vi "DiffDrivePoseEst2_Execute.vi"(0 "Vision TImeStamp_Seconds":dbl=0.02, 3 "TrackWidth_Meters":dbl=1.2 format="%#_13g", 4 "visionRobotPose":T1={"TRANSLATION"={"X"=0.0, "Y"=0.0}, "ROTATION"={"VALUE"=0.0, "COS"=1.0, "SIN"=0.0}} {"ROTATION"."SIN" format="%13.4f"; "ROTATION"."COS" format="%13.4f"; "ROTATION"."VALUE" format="%13.4f"; "TRANSLATION"."Y" format="%14.3f"; "TRANSLATION"."X" format="%14.3f"}, 5 "Game Started":bool, 6 "Add Vision Meas":bool, 7 "InitialPose":T1={"TRANSLATION"={"X"=0.0, "Y"=0.0}, "ROTATION"={"VALUE"=0.0, "COS"=1.0, "SIN"=0.0}} {"ROTATION"."SIN" format="%13.4f"; "ROTATION"."COS" format="%13.4f"; "ROTATION"."VALUE" format="%13.4f"; "TRANSLATION"."Y" format="%14.3f"; "TRANSLATION"."X" format="%14.3f"}, 8 "Pass Through Time":dbl=-1.0, 9 "Gyro Degrees":dbl, 10 "RightDistance_M":dbl=0.02, 11 "LeftDistance_M":dbl=0.02) -> (1 "Error":bool, 2 "Estimated Pose":T1={"TRANSLATION"={"X"=0.0, "Y"=0.0}, "ROTATION"={"VALUE"=0.0, "COS"=1.0, "SIN"=0.0}} {"ROTATION"."SIN" format="%13.4f"; "ROTATION"."COS" format="%13.4f"; "ROTATION"."VALUE" format="%13.4f"; "TRANSLATION"."Y" format="%14.3f"; "TRANSLATION"."X" format="%14.3f"})   [LabVIEW 2020]
uses:
  <vilib>/Rock Robotics/WPI/ThirdParty/JAS_Junk/TrajLib/TypeDef/POSE2D.ctl
  <vilib>/Rock Robotics/WPI/ThirdParty/JAS_Junk/TrajLib/TypeDef/TRANSLATION2D.ctl
  <vilib>/Rock Robotics/WPI/ThirdParty/JAS_Junk/TrajLib/TypeDef/ROTATION2D.ctl
  <vilib>/Rock Robotics/WPI/ThirdParty/JAS_Junk/TrajLib/Conv_Deg_Radians.vi
  <vilib>/Rock Robotics/WPI/ThirdParty/JAS_Junk/TrajLib/Rotation2d_CreateAngle.vi
  <vilib>/Rock Robotics/WPI/ThirdParty/JAS_Junk/TrajLib/VI/Util_GetTime_U32.vi
  <vilib>/Rock Robotics/SystemInterfaces/NetworkCommunication/NetComm_UsageReport_report.vi
  <vilib>/Rock Robotics/WPI/ThirdParty/JAS_Junk/TrajLib/VI/Util_GetTime_U64.vi
  <vilib>/Rock Robotics/WPI/ThirdParty/JAS_Junk/TrajLib/Globals/Util_LibraryGlobals.vi
  <vilib>/Rock Robotics/WPI/ThirdParty/JAS_Junk/TrajLib/Trajectory_Library.lvlib
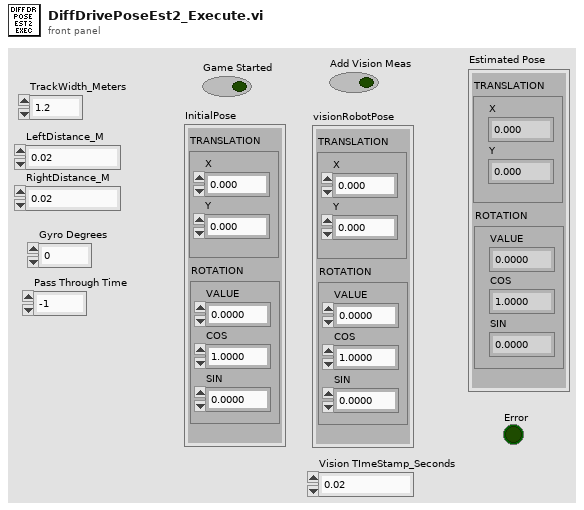
[diagram p1: front panel]
types:
  T1 = typedef "Trajectory_Library.lvlib/POSE2D.ctl" = cluster{"TRANSLATION":T2, "ROTATION":T3}
  T2 = typedef "Trajectory_Library.lvlib/TRANSLATION2D.ctl" = cluster{"X":dbl, "Y":dbl}
  T3 = typedef "Trajectory_Library.lvlib/ROTATION2D.ctl" = cluster{"VALUE":dbl, "COS":dbl, "SIN":dbl}
  T4 = typedef "Trajectory_Library.lvlib/DIFF_DRIVE_KINEMATICS.ctl" = cluster{"TrackWidth_Meters":dbl}
  T5 = typedef "Trajectory_Library.lvlib/DIFF_DRIVE_POSE_EST2.ctl" = cluster{"M_Vision_K":T6, "m_nominal_dT":dbl, "m_PrevTime_Sec":dbl, "Pose_Buffer":T7, "Diff_Drive_Kinematics":T4, "Diff_Drive_Odom_2":T8, "M_Q":T6}
  T6 = typedef "NI_Matrix.lvlib/RealMatrix.ctl" = dbl[][]
  T7 = typedef "Trajectory_Library.lvlib/TIME_INTERPOLATABLE_VARIANT.ctl" = cluster{"TimeStamps":dbl[], "DataArray":variant[], "Min_TimeStamp":dbl, "Max_TimeStamp":dbl, "ItemCount":i32, "MaxBufferTime":dbl}
  T8 = typedef "Trajectory_Library.lvlib/DIFF_DRIVE_ODOM2.ctl" = cluster{"M_POSE_Meters":T1, "M_GyroOffset":T3, "M_PrevAngle":T3, "M_PrevLeftDist_M":dbl, "M_PrevRightDist_M":dbl, "M_InitLeftDist_M":dbl, "M_InitRightDist_M":dbl}
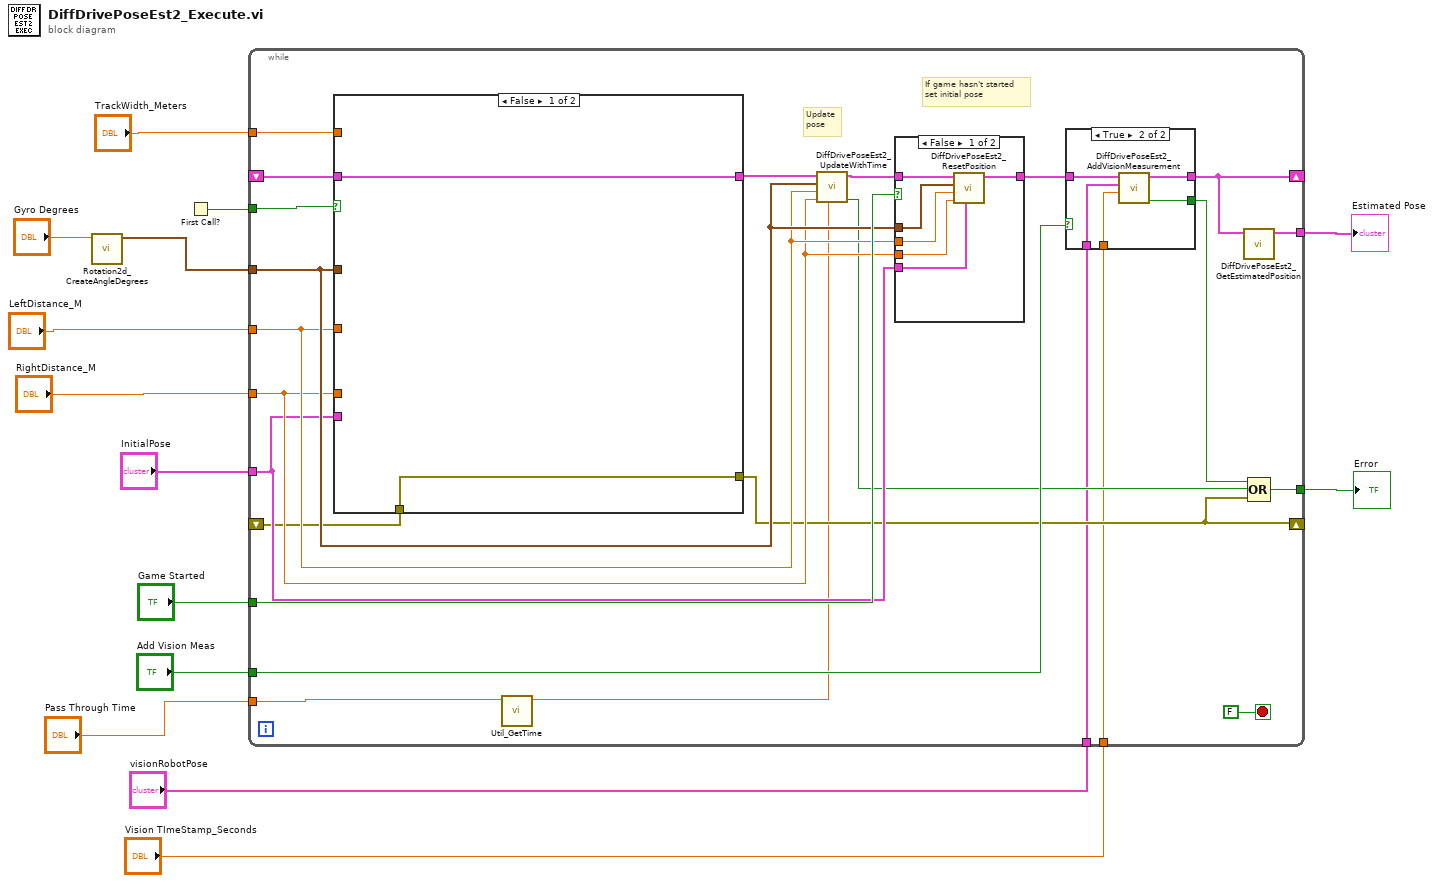
[diagram p0: block diagram]
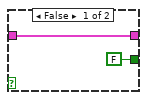
[diagram p3: hidden frame]
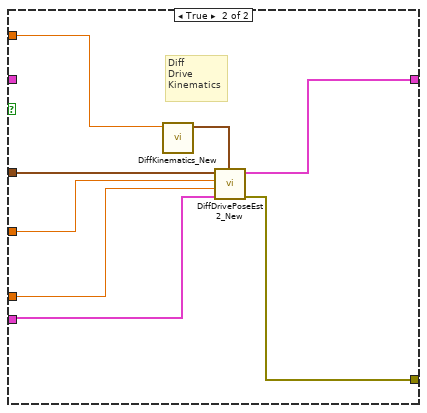
[diagram p4: hidden frame]
diagram:
  n1 = call <vilib>:"Rotation2d_CreateAngleDegrees.vi"("Angle_Degrees"="Gyro Degrees") -> ("ROTATION"=w3:T3)  [unwired: 10 in]
  n2 = First Call?() -> (First Call?: T/F=w14:bool)
  n3 = while {
    tunnel: w14 -> [w37]
    tunnel: w3 -> [w33]
    tunnel: "LeftDistance_M" -> [w32]
    tunnel: "RightDistance_M" -> [w31]
    tunnel: "InitialPose" -> [w30]
    tunnel: "Game Started" -> [w34]
    shift-right: [w23] -> _
    shift-left: _ -> [w28]
    tunnel: "Add Vision Meas" -> [w27]
    shift-right: [w24] -> _
    shift-left: _ -> [w18]
    tunnel: [w22] -> w8
    tunnel: [w21] -> w7
    tunnel: "visionRobotPose" -> [w20]
    tunnel: "Vision TImeStamp_Seconds" -> [w19]
    tunnel: "Pass Through Time" -> [w16]
    tunnel: "TrackWidth_Meters" -> [w15]
    stop <- FALSE stop-if-true
    # "If game hasn't started\nset initial pose"
    # "Update\npose"
    n4 = case shown="False" w37 {
      tunnel: w33 -> [_ w61]
      tunnel: w32 -> [_ w60]
      tunnel: w31 -> [_ w59]
      tunnel: w30 -> [_ w58]
      tunnel: [w53 w57] -> w24
      tunnel: [w54 w56] -> w36
      tunnel: w28 -> [w54 _]
      tunnel: w18 -> [w53 _]
      tunnel: w15 -> [_ w55]
      frame False {
      }
      frame True {
        # "Diff\nDrive\nKinematics"
        n5 = call <vilib>:"DiffKinematics_New.vi"("TrackWidth_Meters"=w55) -> ("DIFF_DRIVE_KINEMATICS"=w62:T4)  [unwired: 10 in]
        n6 = call <vilib>:"DiffDrivePoseEst2_New.vi"("DIFF_DRIVE_KINEMATICS"=w62, "InitialPose"=w58, "RightDistance_M"=w59, "LeftDistance_M"=w60, "gyroAngle"=w61) -> ("Error"=w57:errorcluster, "DiffDrivePoseEstimate"=w56:T5)  [unwired: 5 in]
      }
    }
    n7 = call <vilib>:"Util_GetTime.vi"("Pass_Through_Time"=w16) -> ("FPGA_Time_Seconds"=w17:dbl)  [unwired: 8 in, 2 out]
    n8 = call <vilib>:"DiffDrivePoseEst2_UpdateWithTime.vi"("CurrentTimeSeconds"=w17, "RightDistance"=w31, "LeftDistance"=w32, "GyroAngle"=w33, "in DiffDrivePoseEst2"=w36) -> ("Error"=w26:bool, "Out DiffDrivePoseEst2"=w35:T5)  [unwired: 4 in, 1 out]
    n9 = case shown="False" w34 {
      tunnel: w35 -> [w44 w45]
      tunnel: w33 -> [w43 _]
      tunnel: w32 -> [w42 _]
      tunnel: w31 -> [w41 _]
      tunnel: w30 -> [w40 _]
      tunnel: [w39 w45] -> w29
      frame False {
        n10 = call <vilib>:"DiffDrivePoseEst2_ResetPosition.vi"("Pose"=w40, "RightDistance_M"=w41, "LeftDistance_M"=w42, "Gyro"=w43, "in DiffDrivePoseEst2"=w44) -> ("Out DiffDrivePoseEst2"=w39:T5)  [unwired: 6 in]
      }
      frame True {
      }
    }
    n11 = case shown="True" w27 {
      tunnel: w29 -> [w47 w52]
      tunnel: [w47 w51] -> w23
      tunnel: [FALSE ("Error") w50] -> w25
      tunnel: w20 -> [_ w49]
      tunnel: w19 -> [_ w48]
      frame False {
      }
      frame True {
        n12 = call <vilib>:"DiffDrivePoseEst2_AddVisionMeasurement.vi"("TImeStamp_Seconds"=w48, "visionRobotPose"=w49, "in DiffDrivePoseEst2"=w52) -> ("Error"=w50:bool, "Out DiffDrivePoseEst2"=w51:T5)  [unwired: 7 in]
      }
    }
    n13 = call <vilib>:"DiffDrivePoseEst2_GetEstimatedPosition.vi"("in DiffDrivePoseEstimate"=w23) -> ("Estimated Pose"=w22:T1)  [unwired: 10 in]
    n14 = Compound Arithmetic op=OR(w25, w26, w24) -> (w21:bool)
  }
  "Estimated Pose" <- w8
  "Error" <- w7
